vi "AO DAQ.vi"(11 "Queue ref":T1) -> ()   [LabVIEW 2022 SP3]
uses:
  Controls/All Queue.ctl
  Controls/DAQ case.ctl
  Controls/UI Data.ctl
  Controls/All Loop Status.ctl
  <vilib>/DAQmx/write.llb/DAQmx Write (Analog 1D DBL NChan 1Samp).vi
  Create Task/AO Create Task.vi
  Sub VI's/Global 1.vi
  <vilib>/DAQmx/miscellaneous.llb/DAQmx Fill In Error Info.vi
panel:
  # "TC channel list"
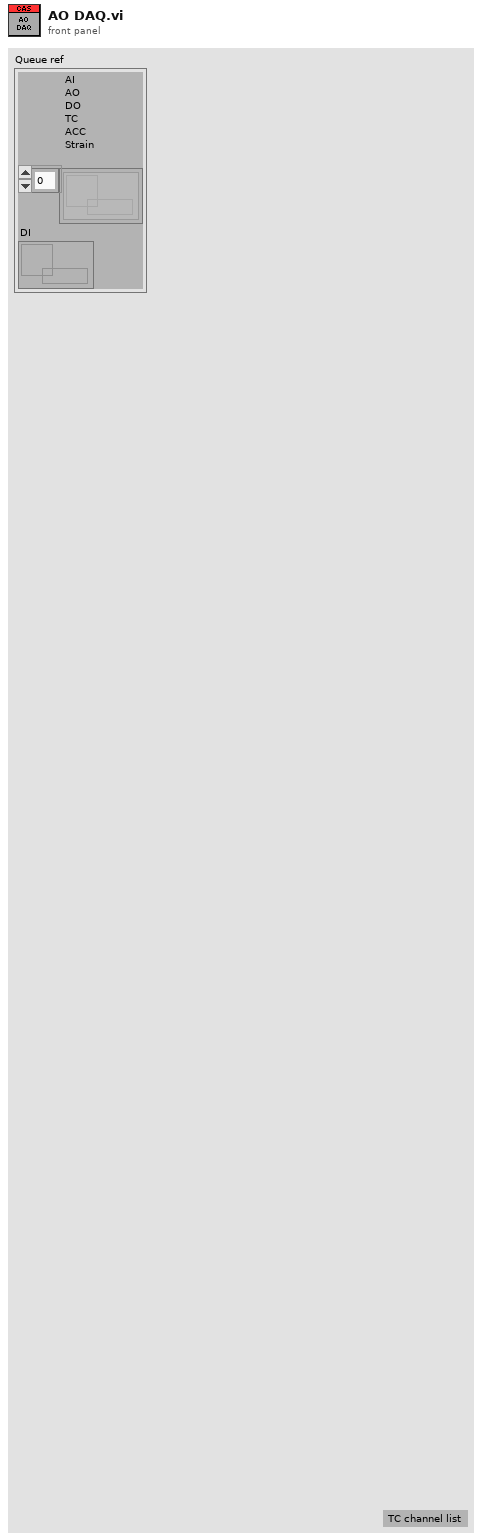
[diagram p1: front panel]
types:
  T1 = typedef "All Queue.ctl" = cluster{"AI\nAO\nDO\nTC\nACC\nStrain":refnum<queue>[], "DI":refnum<queue>}
  T2 = cluster{"in progress?":bool, "Start DAQ":refnum<notifier>, "UI Data":refnum<notifier>, "task out":refnum<k21>, "AO Ref":refnum<queue>, "Loop Rate":u32}
  T3 = typedef "DAQ case.ctl" = enum16{"Initailise", "Create Task", "Polevent", "Acquire", "Stop DAQ", "Error", "Exit"}
  T4 = typedef "All Loop Status.ctl" = enum16{"AI", "AO", "DI", "DO", "TC", "Strain", "ACC", "RT", "Log"}
  T5 = enum16{"Init", "Read 'All'", "Read 'n'", "Read '1'", "Write '1'", "Write 'n'", "Write 'All'"}
  T6 = typedef "All Notifer.ctl" = cluster{"UI Data":refnum<notifier>, "Start DAQ":refnum<notifier>, "Start Log":refnum<notifier>}
  T7 = cluster{"Analog input":bool, "Analog Output":bool, "Digital input":bool, "Digital output":bool, "Thermocouple":bool, "Strain Gauge":bool, "Accelerometer":bool}
  T8 = typedef "Config.ctl" = cluster{"AO config":cluster{"Channel_Name":string, "Channel_Number":string, "Default_Value":dbl, "Units":string}[], "AI config":cluster{"Channel_Name":string, "Channel_Number":string, "Pre_Scale_min":dbl, "Pre_Scale_max":dbl, "Sensor_min":dbl, "Sensor_max":dbl, "Units":string}[], "DI config":cluster{"Channel_Name":string, "Channel_Number":string, "Default_Value":bool, "DI invert?":bool}[], "DO config":cluster{"Channel_Name":string, "Channel_Number":string, "Default_Value":bool, "DO invert?":bool}[], "TC config":cluster{"Channel_Name":string, "Channel_Number":string, "Pre_Scale_min":dbl, "Pre_Scale_max":dbl, "units":i32, " type":i32}[], "ACC config":cluster{"Channel_Name":string, "Channel_Number":string, "Pre_Scale_min":dbl, "Pre_Scale_max":dbl, "Terminal configuration":i32, "Sensitivity":dbl, "Sensitivity units":i32}[], "SG config":cluster{"Channel_Name":string, "Channel_Number":string, "Pre_Scale_min":dbl, "Pre_Scale_max":dbl}[], "Strain Gauge Settings":cluster{"poisson ratio":dbl, "nominal gage resistance":dbl, "gage factor":dbl}, "bridge information":cluster{"strain configuration":i32, "lead wire resistance":dbl, "initial bridge voltage":dbl, "voltage excitation source":i32, "voltage excitation value":dbl}, "Sample Rate":cluster{"AI Sample Rate":dbl, "AO Sample Rate":dbl, "DI Sample Rate":dbl, "TC Sample Rate":dbl, "DO Sample Rate":dbl, "SG Sample Rate":dbl, "ACC Sample Rate":dbl}}
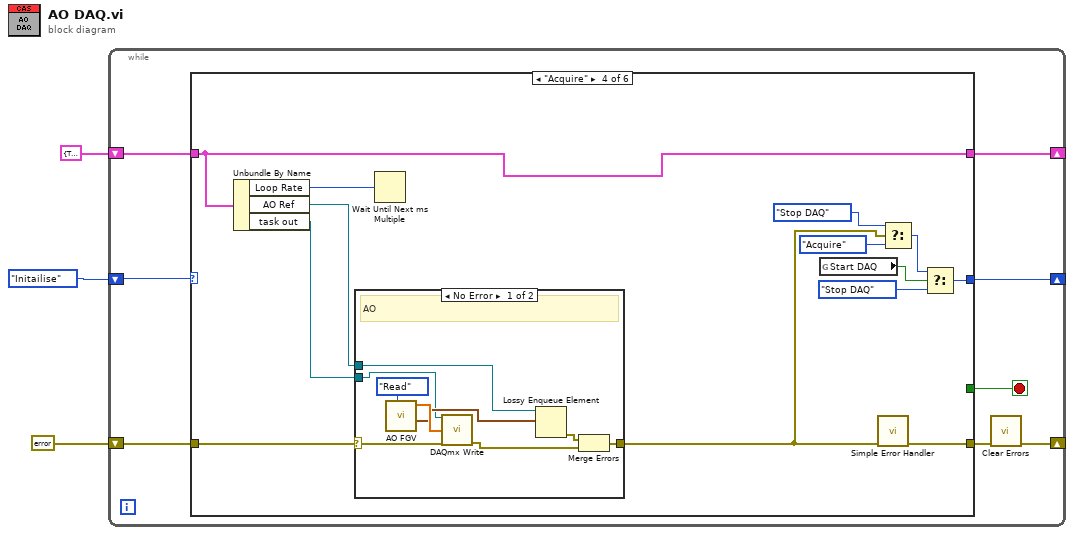
[diagram p0: block diagram]
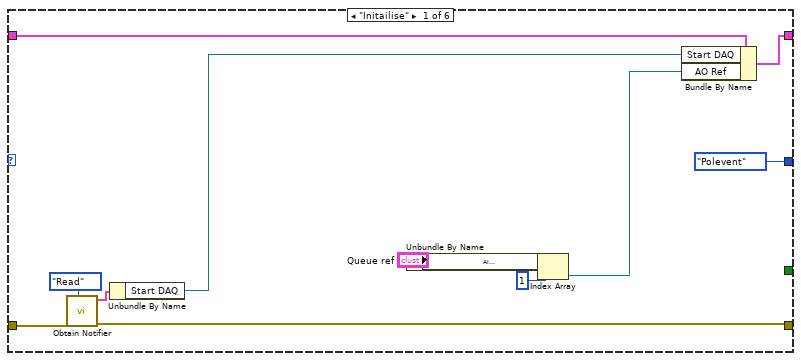
[diagram p2: hidden frame]
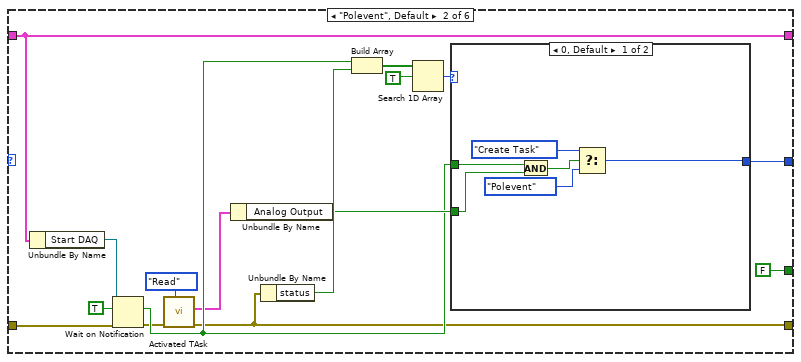
[diagram p3: hidden frame]
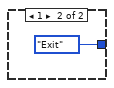
[diagram p4: hidden frame]
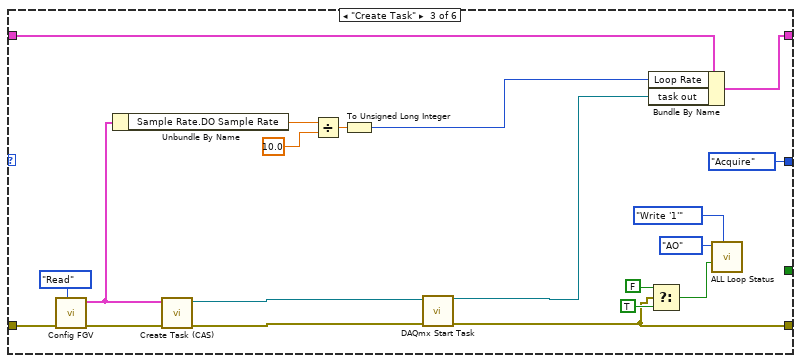
[diagram p5: hidden frame]
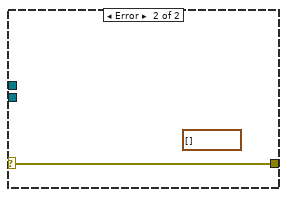
[diagram p6: hidden frame]
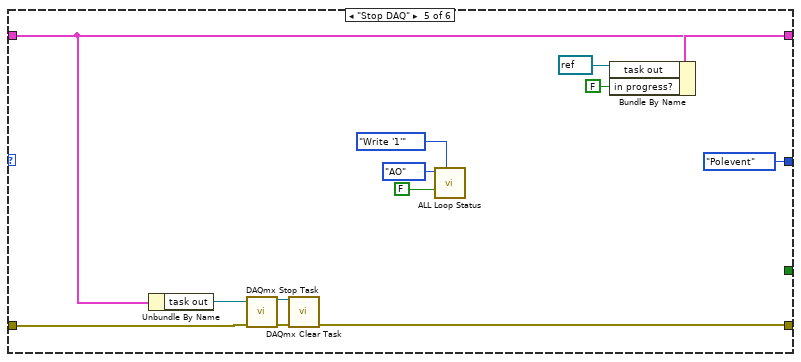
[diagram p7: hidden frame]
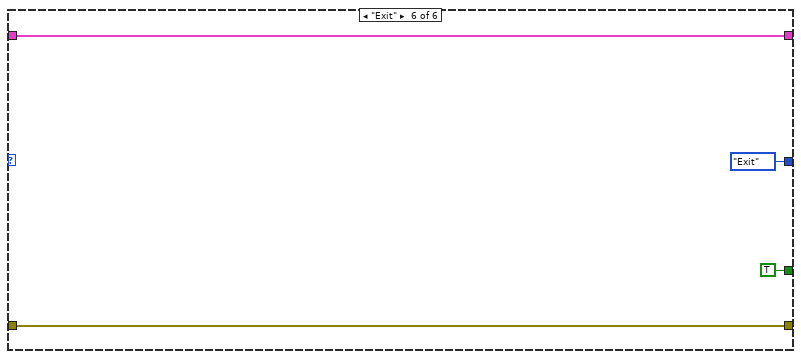
[diagram p8: hidden frame]
diagram:
  n1 = while {
    shift-right: [w4] -> _
    shift-left: errorcluster {"status"=FALSE, "code"=0, "source"=""} ("error out") -> [w10]
    shift-right: [w8] -> _
    shift-left: T2 {"in progress?"=TRUE, "Start DAQ"=refnum, "UI Data"=refnum, "task out"="", "AO Ref"=refnum, "Loop Rate"=0} -> [w9]
    shift-right: [w7] -> _
    shift-left: DAQ_case."Initailise" -> [w6]
    stop <- w11 stop-if-true
    n2 = case shown="\"Acquire\"" w6 {
      tunnel: [_ FALSE _ _ _ TRUE] -> w11
      tunnel: w10 -> [w22 w27 w63 w72 w94 w106]
      tunnel: [w21 w25 w54 w68 w95 w106] -> w5
      tunnel: w9 -> [w19 w37 w65 w73 w99 w105]
      tunnel: [w17 w37 w64 w73 w100 w105] -> w8
      tunnel: [DAQ_case."Polevent" w38 DAQ_case."Acquire" w74 DAQ_case."Polevent" DAQ_case."Exit"] -> w7
      frame "Initailise" {
        n3 = call "Obtain Notifier.vi"("Case"=enum16{"Obtain", "Read"}."Read", "error in (no error)"=w22) -> ("error out"=w21:errorcluster, "notifiers out"=w20:T6)  [unwired: 8 in]
        n4 = Unbundle By Name(w20) -> ("Start DAQ"=w18:refnum<notifier>)
        n5 = Unbundle By Name("Queue ref") -> ("AI\nAO\nDO\nTC\nACC\nStrain"=w14:refnum<queue>[])
        n6 = Index Array(array=w14, index=1) -> (element=w12:refnum<queue>)
        n7 = Bundle By Name(cluster=w19, "Start DAQ"=w18, "AO Ref"=w12) -> (w17:T2)
      }
      frame "Polevent", Default {
        n8 = Unbundle By Name(w37) -> ("Start DAQ"=w36:refnum<notifier>)
        n9 = Wait on Notification(notifier=w36, ignore previous (F)=TRUE, error in (no error)=w27) -> (notification=w28:bool, error out=w26:errorcluster)  [unwired: 1 in, 2 out]
        n10 = call "Activated TAsk.vi"("Enum"=enum16{"Read", "Write"}."Read", "error in (no error)"=w26) -> ("error out"=w25:errorcluster, "Activate Task 2"=w24:T7)  [unwired: 7 in, 1 out]
        n11 = Unbundle By Name(w24) -> ("Analog Output"=w29:bool)
        n12 = Unbundle By Name(w25) -> ("status"=w35:bool)
        n13 = Build Array(w28, w35) -> (w33:bool[])
        n14 = Search 1D Array(1D array=w33, element=TRUE) -> (index of element=w31:i32)  [unwired: 1 in]
        n15 = case shown="0, Default" w31 {
          tunnel: [w44 DAQ_case."Exit"] -> w38
          tunnel: w29 -> [w41 _]
          tunnel: w28 -> [w40 _]
          frame 0, Default {
            n16 = And(x=w40, y=w41) -> (x .and. y?=w42:bool)
            n17 = Select(t=DAQ_case."Create Task", s=w42, f=DAQ_case."Polevent") -> (s? t:f=w44:T3)
          }
          frame 1 {
          }
        }
      }
      frame "Create Task" {
        n18 = call "Config FGV.vi"("Enum"=enum16{"Read", "Write"}."Read", "error in (no error)"=w63) -> ("error out"=w61:errorcluster, "Data"=w51:T8)  [unwired: 8 in]
        n19 = Unbundle By Name(w51) -> ("Sample Rate.DO Sample Rate"=w50:dbl)
        n20 = call-poly "Create Task (CAS).vi"("error in"=w61, "Config"=w51) -> ("error out"=w55:errorcluster, "task out"=w53:refnum<k21>)  [unwired: 7 in, 1 out]
        n21 = Divide(x=w50, y=10.0) -> (x/y=w48:dbl)
        n22 = To Unsigned Long Integer(number=w48) -> (unsigned 32bit integer=w47:u32)
        n23 = call <vilib>:"DAQmx Start Task.vi"("task/channels in"=w53, "error in"=w55) -> ("task out"=w52:refnum<k21>, "error out"=w54:errorcluster)  [unwired: 12 in]
        n24 = Bundle By Name(cluster=w65, "Loop Rate"=w47, "task out"=w52) -> (w64:T2)
        n25 = Select(t=FALSE, s=w54, f=TRUE) -> (s? t:f=w58:bool)
        n26 = call "ALL Loop Status.vi"("Option"=T5."Write '1'", "Status"=w58, "Loop"=All_Loop_Status."AO") -> ()  [unwired: 6 in, 3 out]
      }
      frame "Acquire" {
        n27 = Unbundle By Name(w73) -> ("Loop Rate"=w67:u32, "AO Ref"=w71:refnum<queue>, "task out"=w70:refnum<k21>)
        n28 = case shown="No Error" w72 {
          selector: w72 -> [w85 w89]
          tunnel: w70 -> [w80 _]
          tunnel: [w87 w89] -> w69
          tunnel: w71 -> [w82 _]
          frame No Error {
            # "AO"
            n29 = call "AO FGV.vi"("Enum"=enum16{"Read", "Write", "Start time", "init"}."Read") -> ("AO Waveform"=w81:waveform(dbl)[], "AO out"=w86:dbl[])  [unwired: 9 in]
            n30 = call-poly <vilib>:"DAQmx Write.vi"("task/channels in"=w80, "data"=w86, "error in"=w85) -> ("error out"=w84:errorcluster)  [unwired: 10 in, 2 out]
            n31 = Lossy Enqueue Element(queue=w82, element=w81) -> (error out=w88:errorcluster)  [unwired: 1 in, 3 out]
            n32 = Merge Errors(w88, w84) -> (w87:errorcluster)
          }
          frame Error {
            (unwired) digitalwaveform[] [] ("data")
          }
        }
        n33 = Wait Until Next ms Multiple(millisecond multiple=w67) -> ()  [unwired: 1 out]
        n34 = global read "Global 1.vi" "Start DAQ"() -> (w77:bool)
        n35 = call <vilib>:"Simple Error Handler.vi"("error in (no error)"=w69) -> ("error out"=w68:errorcluster)  [unwired: 4 in, 4 out]
        n36 = Select(t=DAQ_case."Stop DAQ", s=w69, f=DAQ_case."Acquire") -> (s? t:f=w76:T3)
        n37 = Select(t=w76, s=w77, f=DAQ_case."Stop DAQ") -> (s? t:f=w74:T3)
      }
      frame "Stop DAQ" {
        n38 = Unbundle By Name(w99) -> ("task out"=w93:refnum<k21>)
        n39 = call <vilib>:"DAQmx Stop Task.vi"("task/channels in"=w93, "error in"=w94) -> ("task out"=w92:refnum<k21>, "error out"=w96:errorcluster)  [unwired: 12 in]
        n40 = call <vilib>:"DAQmx Clear Task.vi"("task in"=w92, "error in"=w96) -> ("error out"=w95:errorcluster)  [unwired: 13 in]
        n41 = call "ALL Loop Status.vi"("Option"=T5."Write '1'", "Status"=FALSE, "Loop"=All_Loop_Status."AO") -> ()  [unwired: 6 in, 3 out]
        n42 = Bundle By Name(cluster=w99, "task out"=refnum<k21> refnum, "in progress?"=FALSE) -> (w100:T2)
      }
      frame "Exit" {
      }
    }
    n43 = call <vilib>:"Clear Errors.vi"("error in (no error)"=w5) -> ("error out"=w4:errorcluster)  [unwired: 5 in, 1 out]
  }
